vi "Elevator Mode Select.vi"(10 "Manual?":bool, 11 "Auto?":bool) -> (3 "Elevator Mode":T1)   [LabVIEW 2017]
uses:
  Common Code/Elevator Mode.ctl
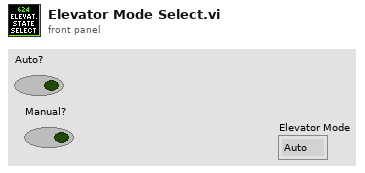
[diagram p1: front panel]
types:
  T1 = typedef "Elevator Mode.ctl" = enum16{"Auto", "Manual"}
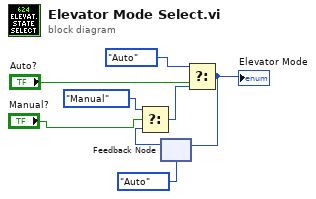
[diagram p0: block diagram]
diagram:
  n1 = feedback #1(enum16{"Auto", "Manual"}."Auto" ("Elevator Mode")) -> (w3:T1)
  n2 = Select(t=enum16{"Auto", "Manual"}."Manual" ("Elevator Mode"), s="Manual?", f=w3) -> (s? t:f=w5:T1)
  n3 = Select(t=Elevator_Mode."Auto" ("Elevator Mode"), s="Auto?", f=w5) -> (s? t:f=w1:T1)
  "Elevator Mode" <- w1
  n4 = feedback-in #1(w1) -> ()
